vi "Step Core.vi"(8 "error in (no error)":errorcluster, 11 "Harmonics in":refnum<class "Harmonics.lvclass">) -> (0 "error out":errorcluster, 3 "Harmonics out":refnum<class "Harmonics.lvclass">)   [LabVIEW 2016, in "Harmonics.lvlib" / "Harmonics.lvclass"]
uses:
  Harmonics.lvclass
  Plugins/Measurement Interface.lvlibp/Measurement Interface.lvclass
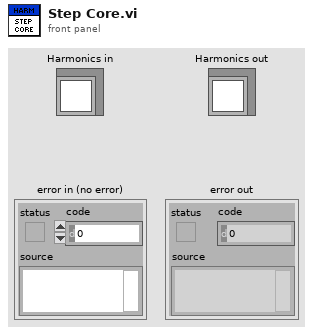
[diagram p1: front panel]
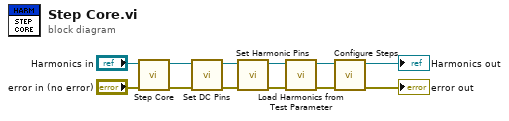
[diagram p0: block diagram]
diagram:
  n1 = call-parent "Step Core.vi"("error in (no error)"="error in (no error)", "Measurement Interface in"="Harmonics in") -> ("error out"=w12:errorcluster, "Measurement Interface out"=w8:refnum<class "Harmonics.lvclass">)  [unwired: 8 in]
  n2 = call "Set DC Pins.vi"("error in (no error)"=w12, "Harmonics in"=w8) -> ("error out"=w9:errorcluster, "Harmonics out"=w6:refnum<class "Harmonics.lvclass">)  [unwired: 8 in]
  n3 = call "Set Harmonic Pins.vi"("error in (no error)"=w9, "Harmonics in"=w6) -> ("error out"=w7:errorcluster, "Harmonics out"=w2:refnum<class "Harmonics.lvclass">)  [unwired: 8 in]
  n4 = call "Load Harmonics from Test Parameter.vi"("error in (no error)"=w7, "Harmonics in"=w2) -> ("error out"=w3:errorcluster, "Harmonics out"=w1:refnum<class "Harmonics.lvclass">)  [unwired: 8 in]
  n5 = call-dynamic "Configure Steps.vi"("error in (no error)"=w3, "Harmonics in"=w1) -> ("error out"=→"error out":errorcluster, "Harmonics out"=→"Harmonics out":refnum<class "Harmonics.lvclass">)  [unwired: 8 in]
